vi "convert_stringlist_to_array.vi"(4 "string list":string) -> (1 "array of strings":string[](array[string]))   [LabVIEW 2017]
doc: "converts a string list (strings separated by comma) to an array of strings\n\nExample:\nstring list: \"plot1, plot2, plot3\""
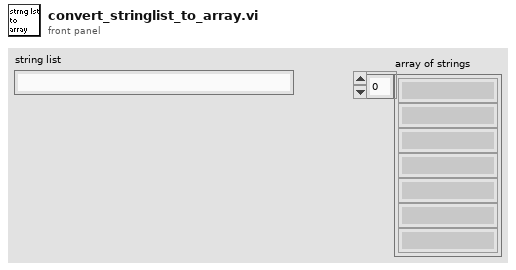
[diagram p1: front panel]
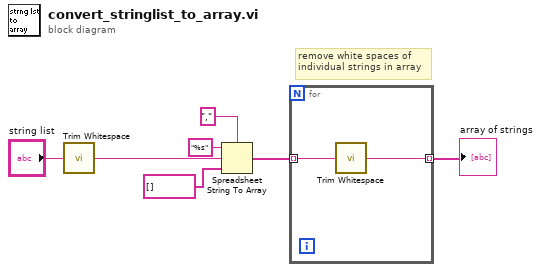
[diagram p0: block diagram]
diagram:
  # "remove white spaces of\nindividual strings in array"
  n1 = call <vilib>:"Trim Whitespace.vi"("string"="string list") -> ("trimmed string"=w6:string)  [unwired: 1 in]
  n2 = Spreadsheet String To Array(delimiter (Tab)=",", format string="%s", spreadsheet string=w6, array type (2D Dbl)=string[] []) -> (array=w2:string[])
  n3 = for {
    tunnel: w2 -> [w9] mode=indexing
    tunnel: [w8] -> w1 mode=indexing
    n4 = call <vilib>:"Trim Whitespace.vi"("string"=w9) -> ("trimmed string"=w8:string)  [unwired: 1 in]
  }
  "array of strings" <- w1
